vi "_UpdatePictureControl.vi"(8 "error in (no error)":errorcluster, 10 "Picture Control Reference":refnum<vi>, 11 "Center Object Reference":refnum<vi>) -> (0 "error out":errorcluster)   [LabVIEW 2017, in "CSM_ExampleBrowser.lvlib"]
uses:
  CSM_ExampleBrowser.lvlib
  <vilib>/Utility/miscctls.llb/LVPointTypeDef.ctl
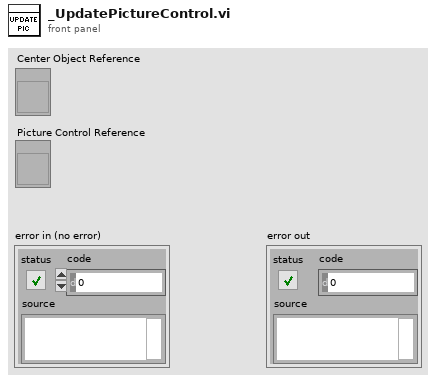
[diagram p1: front panel]
types:
  T1 = typedef "LVPointTypeDef.ctl" = cluster{"Horizontal":i16, "Vertical":i16}
  T2 = typedef "LVRectTypeDef.ctl" = cluster{"Left":i16, "Top":i16, "Right":i16, "Bottom":i16}
  T3 = typedef "LVBoundsTypeDef.ctl" = cluster{"Width":u32, "Height":u32}
  T4 = typedef "imagedata.ctl" = cluster{"image type":i32, "image depth":i32, "image":u8[], "mask":u8[], "colors":u32[], "Rectangle":cluster{"left":i16, "top":i16, "right":i16, "bottom":i16}}
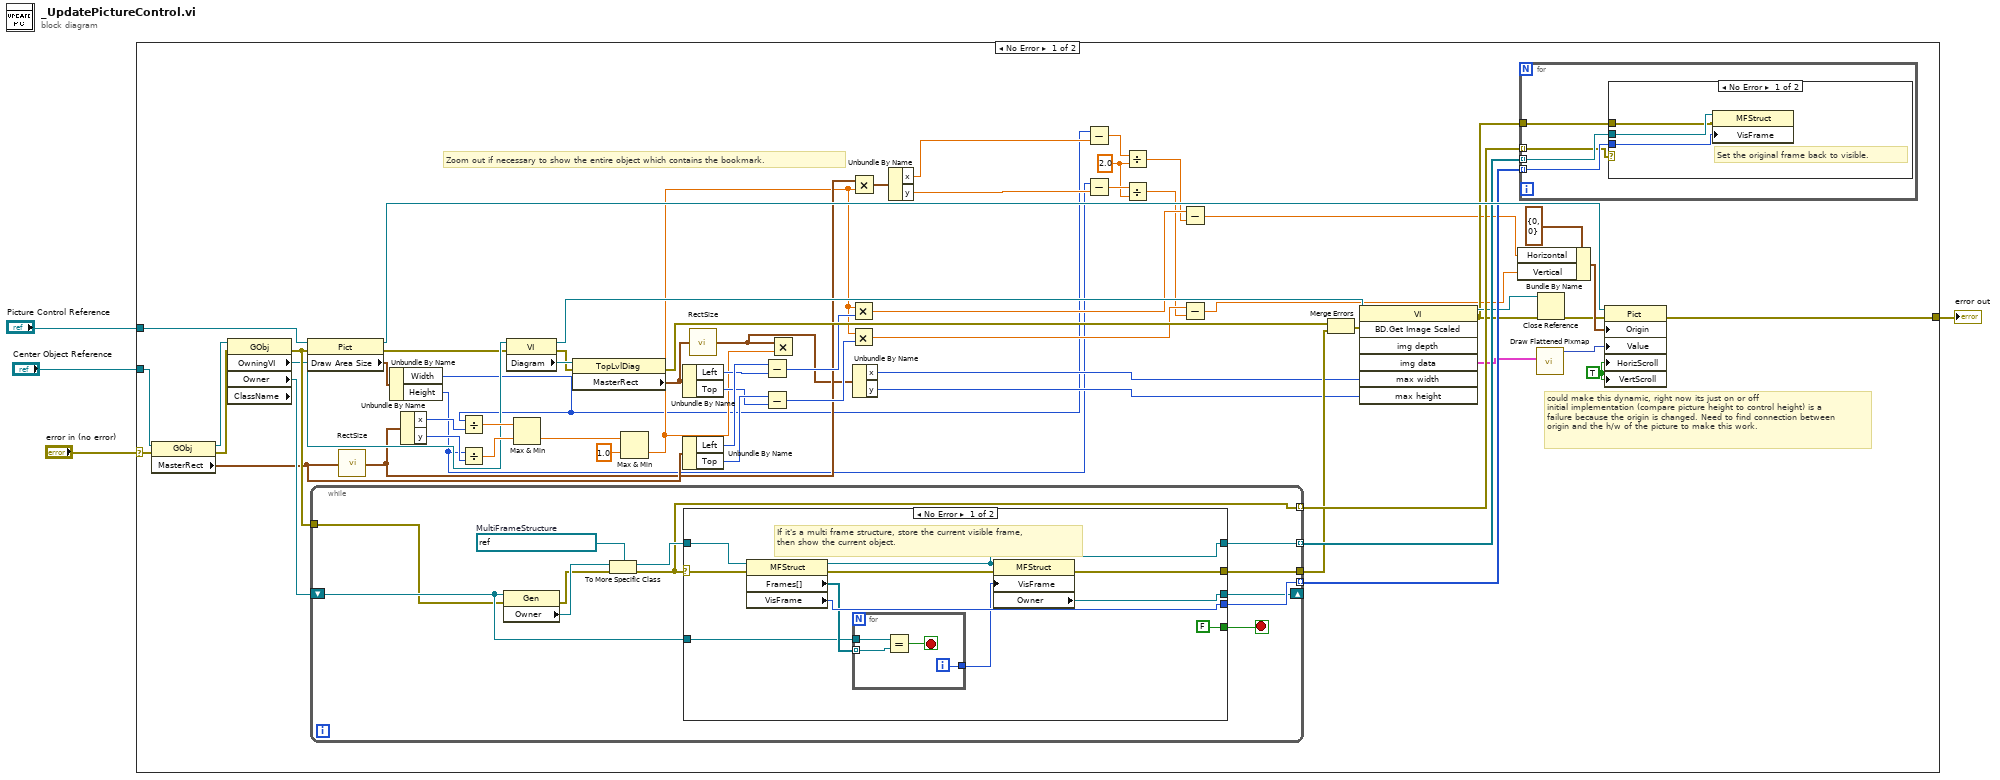
[diagram p0: block diagram]
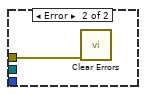
[diagram p2: hidden frame]
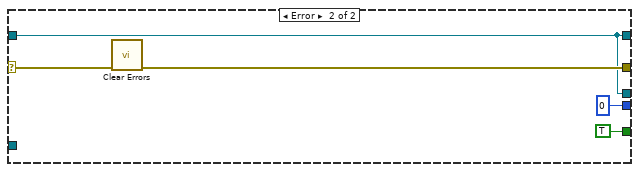
[diagram p3: hidden frame]
diagram:
  n1 = case shown="No Error" "error in (no error)" {
    selector: "error in (no error)" -> [w57 w107]
    tunnel: "Center Object Reference" -> [w62 _]
    tunnel: [w56 w107] -> w2
    tunnel: "Picture Control Reference" -> [w51 _]
    frame No Error {
      w5 = TRUE ("Vertical Scrollbar Visible")
      w18 = 2.0 ("y")
      # "could make this dynamic, right now its just on or off\ninitial implementation (compare picture height to control height) is a failure because the origin is changed. Need to find connection between origin and the h/w of the picture to make this work."
      # "Zoom out if necessary to show the entire object which contains the bookmark."
      n2 = property class="GObj"(reference=w62, error in=w57) -> (reference out=w59:refnum<vi>, error out=w58:errorcluster, "MasterRect"=w26:T2)
      n3 = property class="GObj" props=["OwningVI", "Owner", "ClassName"](reference=w59, error in=w58) -> (error out=w50:errorcluster, "OwningVI"=w44:refnum<vi>, "Owner"=w52:refnum<vi>)  [unwired: 2 out]
      n4 = property class="Pict"(reference=w51, error in=w50) -> (reference out=w60:refnum<vi>, error out=w41:errorcluster, "Draw Area Size"=w45:T3)
      n5 = while {
        tunnel: [w85] -> w55 mode=indexing
        tunnel: [w84] -> w54 mode=indexing
        tunnel: [w82] -> w53 mode=indexing
        tunnel: [w79] -> w39
        tunnel: w50 -> [w77]
        shift-right: [w75] -> _
        shift-left: w52 -> [w78]
        stop <- w76 stop-if-true
        w83 = refnum<vi> refnum  # MultiFrameStructure
        n6 = property class="Gen"(reference=w78, error in=w77) -> (error out=w80:errorcluster, "Owner"=w81:refnum<vi>)  [unwired: 1 out]
        n7 = To More Specific Class(target class=w83, reference=w81, error in=w80) -> (specific class reference=w86:refnum<vi>, error out=w82:errorcluster)
        n8 = case shown="No Error" w82 {
          selector: w82 -> [w91 w106]
          tunnel: w86 -> [w97 w102]
          tunnel: w78 -> [w92 _]
          tunnel: [w89 w105] -> w79
          tunnel: [w96 u32 0 ("VisFrame")] -> w85
          tunnel: [w93 w102] -> w84
          tunnel: [FALSE TRUE] -> w76
          tunnel: [w87 w102] -> w75
          frame No Error {
            # "If it's a multi frame structure, store the current visible frame,\nthen show the current object."
            n9 = property class="MFStruct"(reference=w97, error in=w91) -> (reference out=w93:refnum<vi>, error out=w90:errorcluster, "Frames[]"=w95:refnum<vi>[], "VisFrame"=w96:u32)
            n10 = for {
              tunnel: w95 -> [w101] mode=indexing
              tunnel: w92 -> [w100]
              tunnel: [w98] -> w94
              i -> [w98]
              stop <- w99 stop-if-true
              n11 = Equal?(x=w100, y=w101) -> (x = y?=w99:bool)
            }
            n12 = property class="MFStruct"(reference=w93, error in=w90, "VisFrame"=w94) -> (error out=w89:errorcluster, "Owner"=w87:refnum<vi>)  [unwired: 1 out]
          }
          frame Error {
            n13 = call <vilib>:"Clear Errors.vi"("error in (no error)"=w106) -> ("error out"=w105:errorcluster)  [unwired: 5 in, 1 out]
          }
        }
      }
      n14 = call <vilib>:"RectSize.vi"("rect"=w26) -> ("point"=w25:cluster{"x":i16, "y":i16})
      n15 = Unbundle By Name(w45) -> ("Width"=w8:u32, "Height"=w7:u32)
      n16 = Unbundle By Name(w25) -> ("x"=w49:i16, "y"=w48:i16)
      n17 = Divide(x=w8, y=w49) -> (x/y=w47:dbl)
      n18 = Divide(x=w7, y=w48) -> (x/y=w46:dbl)
      n19 = property class="VI"(reference=w44, error in=w41) -> (reference out=w43:refnum<vi>, error out=w61:errorcluster, "Diagram"=w66:refnum<vi>)
      n20 = Max & Min(x=w47, y=w46) -> (min(x,y)=w35:dbl)  [unwired: 1 out]
      n21 = property class="TopLvlDiag"(reference=w66, error in=w61) -> (error out=w40:errorcluster, "MasterRect"=w27:T2)  [unwired: 1 out]
      n22 = Max & Min(x=w35, y=1.0) -> (min(x,y)=w24:dbl)  [unwired: 1 out]
      n23 = Unbundle By Name(w27) -> ("Left"=w32:i16, "Top"=w29:i16)
      n24 = Unbundle By Name(w26) -> ("Left"=w33:i16, "Top"=w31:i16)
      n25 = call <vilib>:"RectSize.vi"("rect"=w27) -> ("point"=w6:cluster{"x":i16, "y":i16})
      n26 = Subtract(x=w33, y=w32) -> (x-y=w30:i16)
      n27 = Subtract(x=w31, y=w29) -> (x-y=w28:i16)
      n28 = Multiply(x=w6, y=w24) -> ()  [unwired: 1 out]
      n29 = Multiply(x=w24, y=w30) -> (x*y=w17:dbl)
      n30 = Multiply(x=w24, y=w28) -> (x*y=w14:dbl)
      n31 = Multiply(x=w25, y=w24) -> (x*y=w23:cluster{"x":dbl, "y":dbl})
      n32 = Unbundle By Name(w6) -> ("x"=w10:i16, "y"=w9:i16)
      n33 = Unbundle By Name(w23) -> ("x"=w22:dbl, "y"=w20:dbl)
      n34 = Subtract(x=w8, y=w22) -> (x-y=w21:dbl)
      n35 = Subtract(x=w7, y=w20) -> (x-y=w19:dbl)
      n36 = Divide(x=w21, y=w18) -> (x/y=w16:dbl)
      n37 = Divide(x=w19, y=w18) -> (x/y=w13:dbl)
      n38 = Subtract(x=w17, y=w16) -> (x-y=w15:dbl)
      n39 = Subtract(x=w14, y=w13) -> (x-y=w12:dbl)
      n40 = Merge Errors(w40, w39) -> (w38:errorcluster)
      n41 = invoke class="VI" method="BD.Get Image Scaled"(reference=w43, error in=w38, "max width"=w10, "max height"=w9) -> (reference out=w42:refnum<vi>, error out=w37:errorcluster, "img data"=w11:T4)  [unwired: 3 in, 4 out]
      n42 = Bundle By Name(cluster=T1 {"Horizontal"=0, "Vertical"=0} ("Origin"), "Horizontal"=w15, "Vertical"=w12) -> (w63:T1)
      n43 = for {
        tunnel: w55 -> [w70] mode=indexing
        tunnel: w54 -> [w69] mode=indexing
        tunnel: w37 -> [w68]
        tunnel: w53 -> [w67] mode=indexing
        n44 = case shown="No Error" w67 {
          tunnel: w70 -> [w73 _]
          tunnel: w69 -> [w72 _]
          tunnel: w68 -> [w71 w74]
          frame No Error {
            # "Set the original frame back to visible."
            n45 = property class="MFStruct"(reference=w72, error in=w71, "VisFrame"=w73) -> ()  [unwired: 2 out]
          }
          frame Error {
            n46 = call <vilib>:"Clear Errors.vi"("error in (no error)"=w74) -> ()  [unwired: 5 in, 2 out]
          }
        }
      }
      n47 = call <vilib>:"Draw Flattened Pixmap.vi"("image data"=w11) -> ("new picture"=w65:picture)  [unwired: 8 in]
      n48 = Close Reference(reference=w42, error in (no error)=w37) -> (error out=w36:errorcluster)
      n49 = property on="Property Node" class="Pict"(reference=w60, error in=w36, "Origin"=w63, "Value"=w65, "HorizScroll"=w5, "VertScroll"=w5) -> (error out=w56:errorcluster)  [unwired: 1 out]
    }
    frame Error {
    }
  }
  "error out" <- w2
